vi "AutoSetUpMetodo.vi"(8 "error in (no error)":errorcluster, 11 "TektroniksTDS in":refnum<class "TektroniksTDS.lvclass">) -> (0 "error out":errorcluster, 3 "TektroniksTDS out":refnum<class "TektroniksTDS.lvclass">)   [LabVIEW 2020, in "TektroniksTDS.lvclass"]
uses:
  TektroniksTDS.lvclass
  TektroniksTDS.lvclass/TektroniksTDS.ctl
  <instrlib>/Tektronix TDS 200 1000 2000 Series/Tektronix TDS 200 1000 2000 Series.lvlib
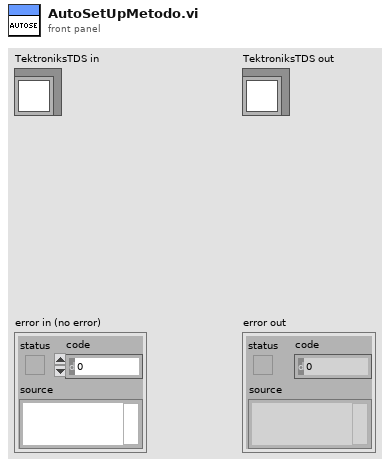
[diagram p1: front panel]
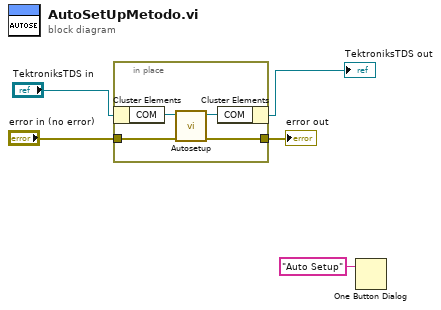
[diagram p0: block diagram]
diagram:
  n1 = in-place {
    in-place-border: "error in (no error)" -> [w8]
    in-place-border: [w7] -> w4
    n2 = in-place-cluster #1("TektroniksTDS in") -> ("COM"=w6:refnum<visa-resource-name>)
    n3 = call <instrlib>:"Autosetup.vi"("error in (no error)"=w8, "VISA resource name"=w6) -> ("error out"=w7:errorcluster, "VISA resource name out"=w9:refnum<visa-resource-name>)  [unwired: 8 in]
    n4 = in-place-cluster #1("COM"=w9) -> (→"TektroniksTDS out":refnum<class "TektroniksTDS.lvclass">)
  }
  "error out" <- w4
  n5 = One Button Dialog(message="Auto Setup") -> ()  [unwired: 1 in, 1 out]
